vi "Subscribe to Results.vi"(8 "error in (no error)":errorcluster, 10 "Result Observer":refnum<class "Result Observer.lvclass">, 11 "LUnit Test Suite In":refnum<class "LUnit Test Suite.lvclass">) -> (0 "error out":errorcluster, 3 "LUnit Test Suite Out":refnum<class "LUnit Test Suite.lvclass">)   [LabVIEW 2020, in "LUnit Test Suite.lvclass"]
uses:
  LUnit Test Suite.lvclass
  Core/Result Observer/Result Observer.lvclass
  LUnit Test Suite.lvclass/LUnit Test Suite.ctl
  Core/Runnable/Runnable.lvclass
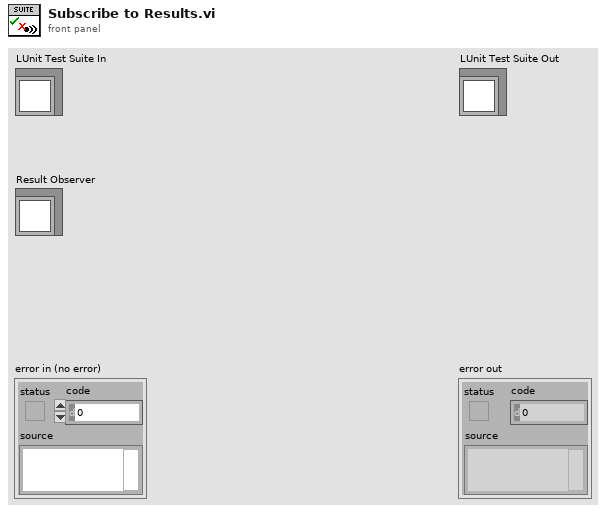
[diagram p1: front panel]
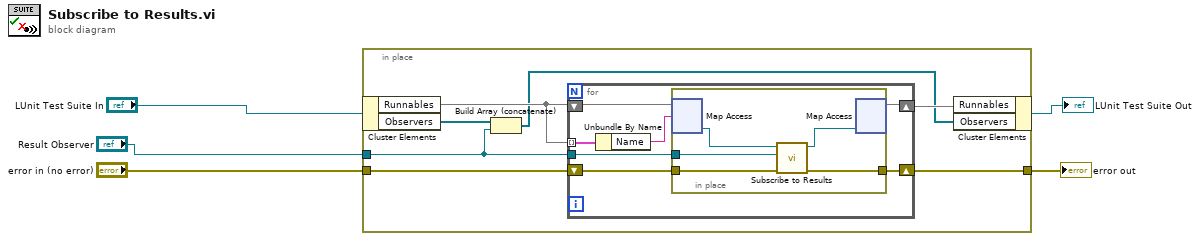
[diagram p0: block diagram]
diagram:
  n1 = in-place {
    in-place-border: "Result Observer" -> [w7]
    in-place-border: "error in (no error)" -> [w12]
    in-place-border: [w11] -> w3
    n2 = in-place-cluster #1("LUnit Test Suite In") -> ("Runnables"=w10:map{string, refnum<class "Runnable.lvclass">}, "Observers"=w8:refnum<class "Result Observer.lvclass">[])
    n3 = Build Array (concatenate)(w8, w7) -> (w6:refnum<class "Result Observer.lvclass">[])
    n4 = for {
      tunnel: w10 -> [w19] mode=indexing
      tunnel: w7 -> [w18]
      shift-right: [w16] -> w11
      shift-left: w12 -> [w17]
      shift-right: [w13] -> w9
      shift-left: w10 -> [w14]
      n5 = Unbundle By Name(w19) -> ("Name"=w15:string)
      n6 = in-place {
        in-place-border: w18 -> [w24]
        in-place-border: w17 -> [w23]
        in-place-border: [w22] -> w16
        n7 = in-place-map #2(w14, w15) -> (w21:refnum<class "Runnable.lvclass">)  [unwired: 1 in, 1 out]
        n8 = call-dynamic "Subscribe to Results.vi"("error in (no error)"=w23, "Result Observer"=w24, "Runnable In"=w21) -> ("error out"=w22:errorcluster, "Runnable Out"=w20:refnum<class "Runnable.lvclass">)  [unwired: 7 in]
        n9 = in-place-map #2(w20) -> (w13:map{string, refnum<class "Runnable.lvclass">})  [unwired: 1 in, 2 out]
      }
    }
    n10 = in-place-cluster #1("Runnables"=w9, "Observers"=w6) -> (→"LUnit Test Suite Out":refnum<class "LUnit Test Suite.lvclass">)
  }
  "error out" <- w3
